vi "CAN_setOutput.vi"(8 "error in (no error)":errorcluster, 9 "Output Right":dbl, 10 "Output Left":dbl) -> (0 "error out":errorcluster)   [LabVIEW 2009, in "OWNCAN.lvlib"]
uses:
  OWNCAN.lvlib
  CAN Jaguars Ref.ctl
  CAN/SubVIs/CAN Jaguar Ref.ctl
  CAN/SubVIs/CAN Jaguar Control Mode.ctl
  CAN.lvlib
panel:
  out "CAN Jaguars Ref out":T1
  in  "CAN Jaguars Ref":T1
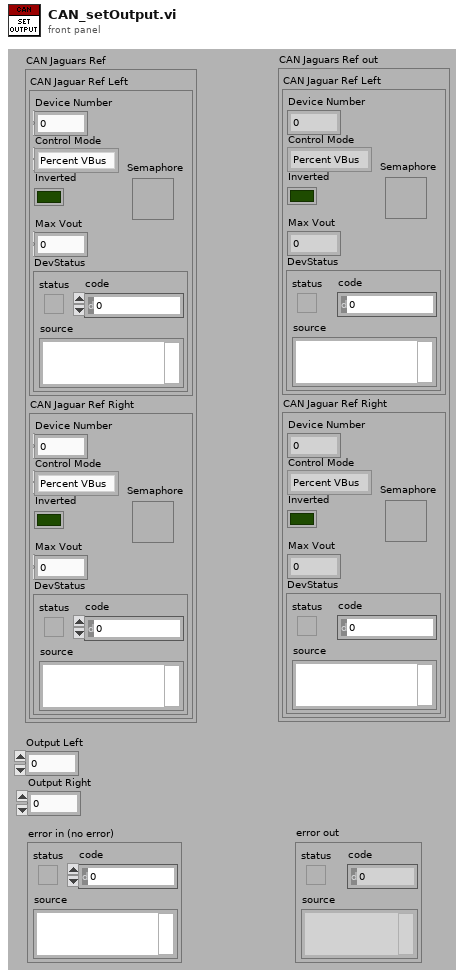
[diagram p1: front panel]
types:
  T1 = typedef "OWNCAN.lvlib/CAN Jaguars Ref.ctl" = cluster{"CAN Jaguar Ref Left":T2, "CAN Jaguar Ref Right":T2}
  T2 = typedef "CAN.lvlib/CAN Jaguar Ref.ctl" = cluster{"Device Number":u8, "Control Mode":T3, "Inverted":bool, "Semaphore":T4, "Max Vout":dbl, "DevStatus":errorcluster}
  T3 = typedef "CAN.lvlib/CAN Jaguar Control Mode.ctl" = enum16{"Percent VBus", "Speed", "Position", "Current"}
  T4 = typedef "Semaphore RefNum" = refnum<k1>
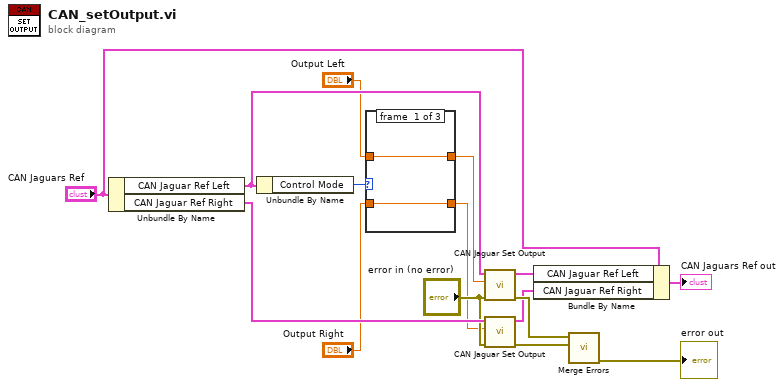
[diagram p0: block diagram]
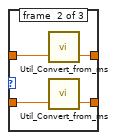
[diagram p2: hidden frame]
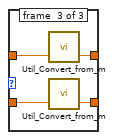
[diagram p3: hidden frame]
diagram:
  n1 = Unbundle By Name("CAN Jaguars Ref") -> ("CAN Jaguar Ref Left"=w10:T2, "CAN Jaguar Ref Right"=w15:T2)
  n2 = Unbundle By Name(w10) -> ("Control Mode"=w9:T3)
  n3 = case shown="\"Percent VBus\", Default" w9 {
    tunnel: "Output Left" -> [w16 w21 w25]
    tunnel: [w16 w20 w24] -> w7
    tunnel: "Output Right" -> [w17 w19 w23]
    tunnel: [w17 w18 w22] -> w5
    frame #0 {
    }
    frame #1 {
      n4 = call "Util_Convert_from_ms.vi"("m/s wheel"=w21) -> ("rpm gear"=w20:dbl)  [unwired: 2 in]
      n5 = call "Util_Convert_from_ms.vi"("m/s wheel"=w19) -> ("rpm gear"=w18:dbl)  [unwired: 2 in]
    }
    frame #2 {
      n6 = call "Util_Convert_from_m.vi"("distance (m) wheel"=w25) -> ("rotations gear"=w24:dbl)  [unwired: 2 in]
      n7 = call "Util_Convert_from_m.vi"("distance (m) wheel"=w23) -> ("rotations gear"=w22:dbl)  [unwired: 2 in]
    }
  }
  n8 = call "CAN Jaguar Set Output.vi"("error in (no error)"="error in (no error)", "Output Set Point"=w7, "CAN Jaguar Ref"=w10) -> ("error out"=w13:errorcluster, "CAN Jaguar Ref Out"=w3:T2)  [unwired: 7 in]
  n9 = call "CAN Jaguar Set Output.vi"("error in (no error)"="error in (no error)", "Output Set Point"=w5, "CAN Jaguar Ref"=w15) -> ("error out"=w14:errorcluster, "CAN Jaguar Ref Out"=w4:T2)  [unwired: 7 in]
  n10 = Bundle By Name(cluster="CAN Jaguars Ref", "CAN Jaguar Ref Left"=w3, "CAN Jaguar Ref Right"=w4) -> (→"CAN Jaguars Ref out":T1)
  n11 = call <vilib>:"Merge Errors.vi"("error in 2 (no error)"=w14, "error in 1 (no error)"=w13) -> ("error out"=→"error out":errorcluster)  [unwired: 5 in]
